vi "Save DUT Information.vi"(8 "error in (no error)":errorcluster, 10 "DUT Info":T1, 11 "csv-formatter in":refnum<class "csv-formatter.lvclass">) -> (0 "error out":errorcluster, 3 "csv-formatter out":refnum<class "csv-formatter.lvclass">)   [LabVIEW 2015, in "csv-formatter.lvclass"]
doc: "This VI will save the DUT Information to the permanent report"
uses:
  csv-formatter.lvclass
  Report Information/DUT Information.ctl
  csv-formatter.lvclass/csv-formatter.ctl
  Report Information/Report Information.lvclass
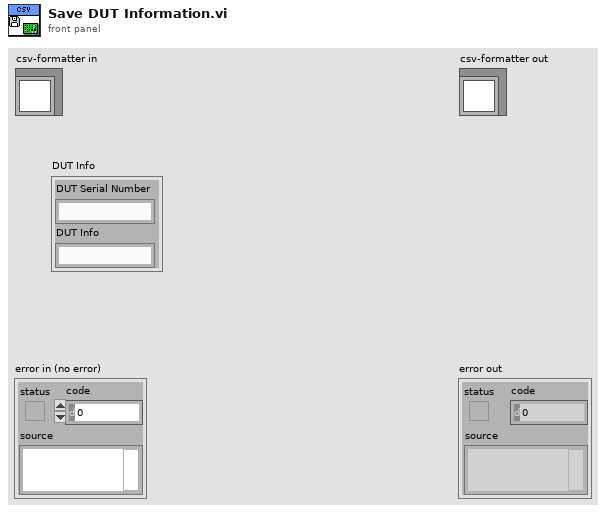
[diagram p1: front panel]
types:
  T1 = typedef "Report Information.lvclass/DUT Information.ctl" = cluster{"DUT Serial Number":string, "DUT Info":string}
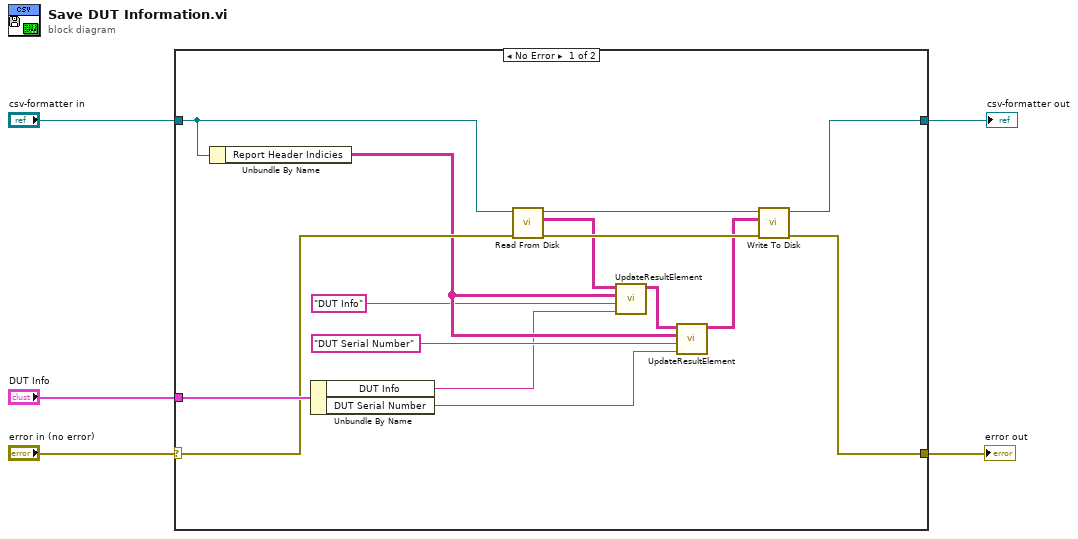
[diagram p0: block diagram]
diagram:
  n1 = case shown="No Error" "error in (no error)" {
    selector: "error in (no error)" -> [w19 w22]
    tunnel: "DUT Info" -> [w20 _]
    tunnel: "csv-formatter in" -> [w16 w21]
    tunnel: [w17 w22] -> w2
    tunnel: [w14 w21] -> w1
    frame No Error {
      n2 = Unbundle By Name(w16) -> ("Report Header Indicies"=w11:string[][])
      n3 = Unbundle By Name(w20) -> ("DUT Info"=w7:string, "DUT Serial Number"=w6:string)
      n4 = call "Read From Disk.vi"("error in (no error)"=w19, "csv-formatter in"=w16) -> ("error out"=w18:errorcluster, "Result Out"=w13:string[][], "csv-formatter out"=w15:refnum<class "csv-formatter.lvclass">)  [unwired: 7 in]
      n5 = call "UpdateResultElement.vi"("Data"=w7, "Lookup String"="DUT Info", "Report Header Indicies in"=w11, "Result in"=w13) -> ("Result Out"=w12:string[][])  [unwired: 6 in, 1 out]
      n6 = call "UpdateResultElement.vi"("Data"=w6, "Lookup String"="DUT Serial Number", "Report Header Indicies in"=w11, "Result in"=w12) -> ("Result Out"=w10:string[][])  [unwired: 6 in, 1 out]
      n7 = call "Write To Disk.vi"("error in (no error)"=w18, "Result In"=w10, "csv-formatter in"=w15) -> ("error out"=w17:errorcluster, "csv-formatter out"=w14:refnum<class "csv-formatter.lvclass">)  [unwired: 7 in]
    }
    frame Error {
    }
  }
  "error out" <- w2
  "csv-formatter out" <- w1
